vi "Init.vi"(8 "error in (no error)":errorcluster, 10 "Connection Info":T1, 11 "FP Manager In":refnum<class "Front Panel Manager.lvclass">) -> (0 "error out":errorcluster, 3 "FP Manager Out":refnum<class "Front Panel Manager.lvclass">)   [LabVIEW 2015, in "Front Panel Publisher.lvlib" / "Front Panel Manager.lvclass"]
uses:
  Front Panel Manager.lvclass
  Controls/Websocket Info.ctl
  Web Front Panel_class/Web Front Panel.lvclass
  Websocket_class/Websocket.lvclass
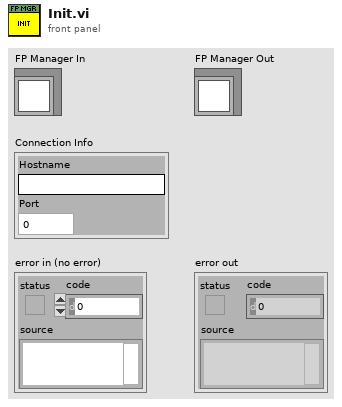
[diagram p1: front panel]
types:
  T1 = typedef "Front Panel Publisher.lvlib/Front Panel Manager.lvclass/Websocket Info.ctl" = cluster{"Hostname":string, "Port":u16}
  T2 = typedef "Front Panel Publisher.lvlib/Front Panel Manager.lvclass/Object Attributes.ctl" = cluster{"WebFrontPanels":refnum<class "Web Front Panel.lvclass">[], "WFP Names":string[], "Root folder":path, "Websocket Info":T1}
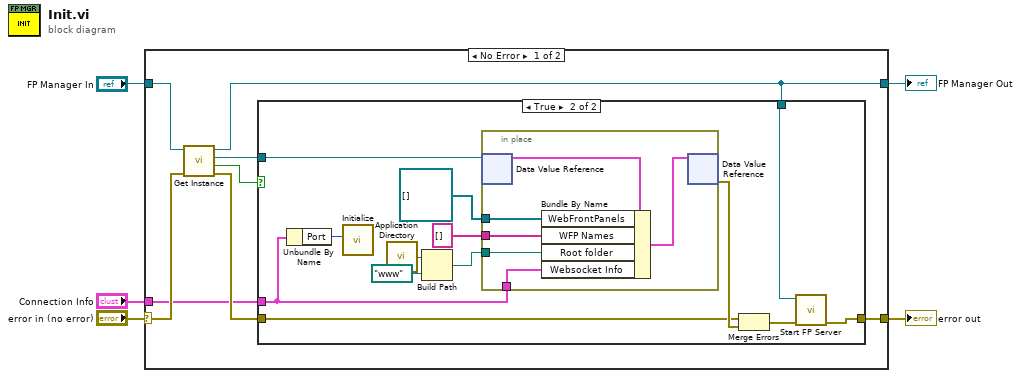
[diagram p0: block diagram]
diagram:
  n1 = case shown="No Error" "error in (no error)" {
    selector: "error in (no error)" -> [w13 w35]
    tunnel: [w6 w35] -> w4
    tunnel: "FP Manager In" -> [w8 w34]
    tunnel: [w7 w34] -> w2
    tunnel: "Connection Info" -> [w9 _]
    frame No Error {
      n2 = call "Get Instance.vi"("error in (no error)"=w13, "FP Manager In"=w8) -> ("error out"=w11:errorcluster, "NewObjectCreated"=w10:bool, "DVRRefOut"=w12:refnum<data-value>, "FP Manager Out"=w7:refnum<class "Front Panel Manager.lvclass">)  [unwired: 5 in, 1 out]
      n3 = case shown="True" w10 {
        tunnel: [w14 w16] -> w6
        tunnel: w12 -> [_ w26]
        tunnel: w11 -> [w14 w20]
        tunnel: w9 -> [_ w19]
        tunnel: w7 -> [_ w15]
        frame False {
        }
        frame True {
          n4 = Unbundle By Name(w19) -> ("Port"=w18:u16)
          n5 = call "Initialize.vi"("Port (81)"=w18) -> ()  [unwired: 9 in, 2 out]
          n6 = call <vilib>:"Application Directory.vi"() -> ("Application Directory"=w22:path)
          n7 = Build Path(base path=w22, name or relative path=path "www") -> (appended path=w21:path)
          n8 = in-place {
            in-place-border: w21 -> [w31]
            in-place-border: string[] [] ("WFP Names") -> [w30]
            in-place-border: refnum<class "Web Front Panel.lvclass">[] [] ("WebFrontPanels") -> [w29]
            in-place-border: w19 -> [w28]
            n9 = in-place-dvr #1(w26) -> (w32:T2)  [unwired: 1 out]
            n10 = Bundle By Name(cluster=w32, "WebFrontPanels"=w29, "WFP Names"=w30, "Root folder"=w31, "Websocket Info"=w28) -> (w33:T2)
            n11 = in-place-dvr #1(w33) -> (w27:errorcluster)  [unwired: 1 out]
          }
          n12 = Merge Errors(w20, w27) -> (w17:errorcluster)
          n13 = call "Start FP Server.vi"("error in (no error)"=w17, "FP Management In"=w15) -> ("error out"=w16:errorcluster)  [unwired: 7 in, 2 out]
        }
      }
    }
    frame Error {
    }
  }
  "error out" <- w4
  "FP Manager Out" <- w2
